vi "Test_ADC.vi"() -> ()   [LabVIEW 2014]
uses:
  <userlib>/UCSD Robotics Lab/Robotics-Cape/LV/libroboticscape.lvlib
panel:
  out "Timing Block":T1 {"Actual Hz" format="%#_3g"; "Dt" format="%#_4g"; "Average Hz" format="%#_4g"}
  out "ADC state":T2
  out "Iteration counter":i32
  out "State":T3(ring)
  in  "stop":bool
  # "Always stop the VI using the rectangular STOP button above, never with the round stopsign (Abort)"
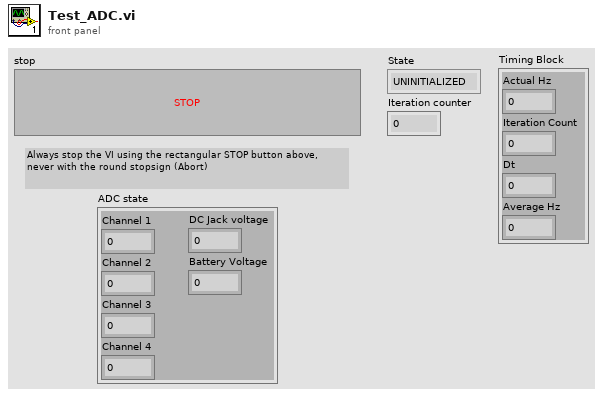
[diagram p1: front panel]
types:
  T1 = cluster{"Actual Hz":dbl, "Iteration Count":dbl, "Dt":dbl, "Average Hz":dbl}
  T2 = cluster{"Channel 1":sgl, "Channel 2":sgl, "Channel 3":sgl, "Channel 4":sgl, "DC Jack voltage":sgl, "Battery Voltage":sgl}
  T3 = enum16{"UNINITIALIZED", "RUNNING", "PAUSED", "EXITING"}
  T4 = enum16{"UNINITIALIZED", "RUNING", "PAUSED", "EXITING"}
  T5 = cluster{"function return":sgl, "function return":sgl, "function return":sgl, "function return":sgl, "function return":sgl, "function return":sgl}
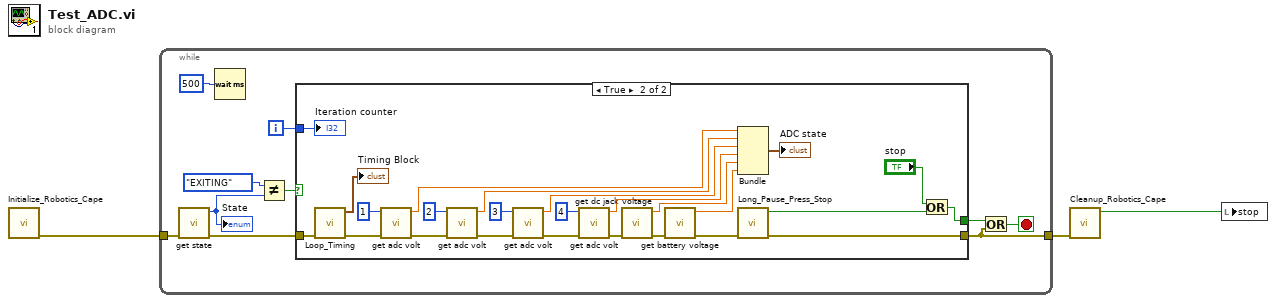
[diagram p0: block diagram]
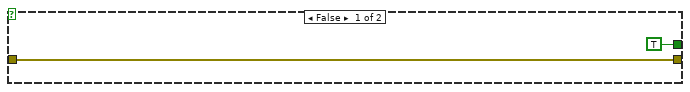
[diagram p2: hidden frame]
diagram:
  n1 = call "Initialize_Robotics_Cape.vi"() -> ("error out"=w3:errorcluster)  [unwired: 11 in]
  n2 = while {
    tunnel: w3 -> [w12]
    tunnel: [w6] -> w2
    i -> [w11]
    stop <- w13 stop-if-true
    n3 = call <userlib>:"get state.vi"("error in (no error)"=w12) -> ("error out"=w7:errorcluster, "function return"=w9:u32)  [unwired: 9 in]
    "State" <- w9
    n4 = Wait (ms)(milliseconds to wait=u32 500) -> ()  [unwired: 1 out]
    n5 = Not Equal?(x=T4."EXITING" ("State 2"), y=w9) -> (x != y?=w8:bool)
    n6 = case shown="True" w8 {
      tunnel: w11 -> [_ w40]
      tunnel: w7 -> [w15 w23]
      tunnel: [w15 w19] -> w6
      tunnel: [TRUE ("stop") w16] -> w5
      frame False {
      }
      frame True {
        n7 = call "Loop_Timing.vi"("error in"=w23) -> ("error out"=w22:errorcluster, "Timing Block"=→"Timing Block":T1)  [unwired: 9 in]
        n8 = call <userlib>:"get adc volt.vi"("error in (no error)"=w22, "ch"=1) -> ("error out"=w35:errorcluster, "function return"=w30:sgl)  [unwired: 8 in]
        n9 = call <userlib>:"get adc volt.vi"("error in (no error)"=w35, "ch"=2) -> ("error out"=w34:errorcluster, "function return"=w29:sgl)  [unwired: 8 in]
        n10 = call <userlib>:"get adc volt.vi"("error in (no error)"=w34, "ch"=3) -> ("error out"=w33:errorcluster, "function return"=w28:sgl)  [unwired: 8 in]
        n11 = call <userlib>:"get adc volt.vi"("error in (no error)"=w33, "ch"=4) -> ("error out"=w32:errorcluster, "function return"=w27:sgl)  [unwired: 8 in]
        n12 = call <userlib>:"get dc jack voltage.vi"("error in (no error)"=w32) -> ("error out"=w31:errorcluster, "function return"=w26:sgl)  [unwired: 9 in]
        n13 = call <userlib>:"get battery voltage.vi"("error in (no error)"=w31) -> ("error out"=w20:errorcluster, "function return"=w25:sgl)  [unwired: 9 in]
        n14 = Bundle("function return"=w30, "function return"=w29, "function return"=w28, "function return"=w27, "function return"=w26, "function return"=w25) -> (→"ADC state":T5)  [unwired: 1 in]
        n15 = call "Long_Pause_Press_Stop.vi"("error in (no error)"=w20) -> ("error out"=w19:errorcluster, "Stop"=w18:bool)  [unwired: 9 in]
        n16 = Or(x="stop", y=w18) -> (x .or. y?=w16:bool)
        "Iteration counter" <- w40
      }
    }
    n17 = Or(x=w5, y=w6) -> (x .or. y?=w13:bool)
  }
  n18 = call "Cleanup_Robotics_Cape.vi"("error in (no error)"=w2) -> ("Stop Local Variabl"=w1:bool)  [unwired: 9 in, 1 out]
  n19 = local write "stop"(w1) -> ()
